vi "BallSequencing.vi"(0 "Balls In Robot":i32, 1 "Speed of Harvester":dbl, 5 "Shoot":bool, 7 "Ball S12 Process":bool, 9 "Ball S3 Process":bool, 11 "Speed of Conveyor":dbl, 12 "SP 1 Triggered":bool, 13 "SP 2 Triggered":bool, 14 "SP 3 Triggered":bool) -> (2 "Conveyer Output":dbl, 3 "Harvester Output":dbl, 4 "Balls In Robot Output":i32, 6 "Shoot Output":bool, 8 "Ball S12 Process Output":bool, 10 "Ball S3 Process Output":bool)   [LabVIEW 2011]
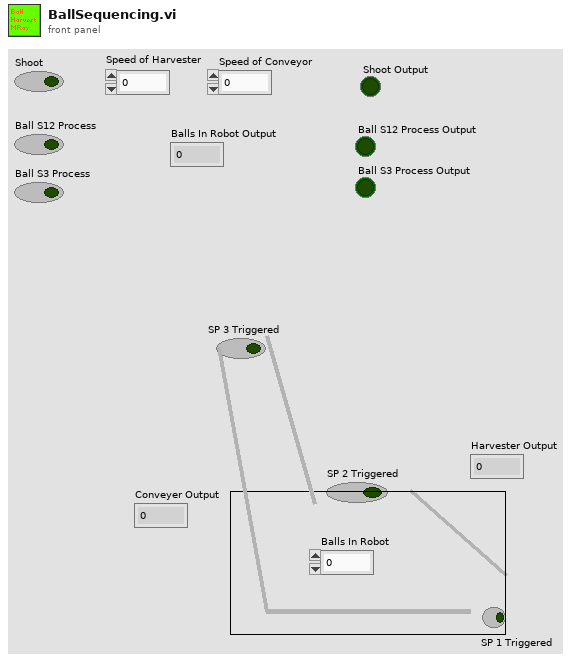
[diagram p1: front panel]
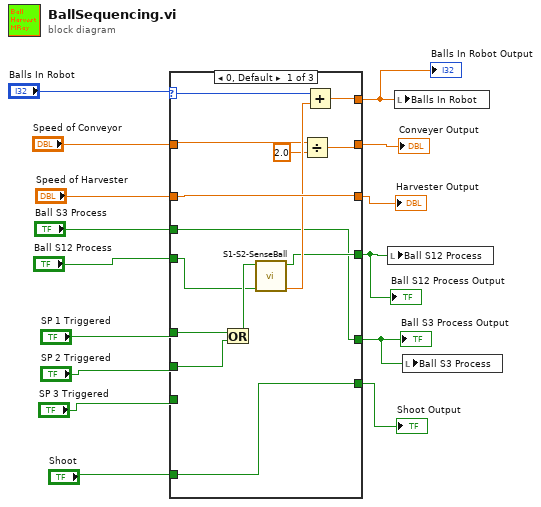
[diagram p0: block diagram]
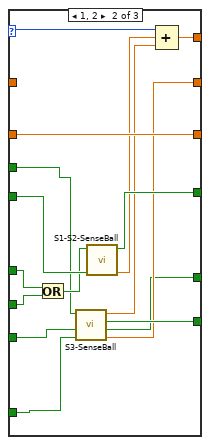
[diagram p2: hidden frame]
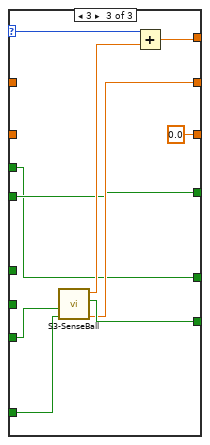
[diagram p3: hidden frame]
diagram:
  n1 = case shown="0, Default" "Balls In Robot" {
    selector: "Balls In Robot" -> [w28 w37 w54]
    tunnel: "SP 1 Triggered" -> [w25 w43 _]
    tunnel: "SP 2 Triggered" -> [w24 w44 _]
    tunnel: [w29 w40 0.0 ("Speed of Harvester")] -> w15
    tunnel: "Speed of Harvester" -> [w29 w40 _]
    tunnel: "Speed of Conveyor" -> [w20 _ _]
    tunnel: [w18 w31 w48] -> w3
    tunnel: [w27 w39 w53] -> w2
    tunnel: "SP 3 Triggered" -> [_ w35 w49]
    tunnel: "Ball S3 Process" -> [w16 w34 w46]
    tunnel: "Ball S12 Process" -> [w22 w45 w47]
    tunnel: [w21 w41 w47] -> w4
    tunnel: "Shoot" -> [w17 w36 w52]
    tunnel: [w17 w33 w51] -> w5
    tunnel: [w16 w30 w46] -> w1
    frame 0, Default {
      n2 = Or(x=w25, y=w24) -> (x .or. y?=w23:bool)
      n3 = call "S1-S2-SenseBall.vi"("Ball in Process in"=w22, "Sense Ball"=w23) -> ("Ball Counter"=w26:dbl, "Ball in Process out"=w21:bool)  [unwired: 8 in]
      n4 = Divide(x=w20, y=2.0) -> (x/y=w18:dbl)
      n5 = Add(x=w28, y=w26) -> (x+y=w27:dbl)
    }
    frame 1, 2 {
      n6 = Or(x=w43, y=w44) -> (x .or. y?=w42:bool)
      n7 = call "S3-SenseBall.vi"("Ball S3 Process"=w34, "Sense Ball"=w35, "Trigger Shooter"=w36) -> ("Ball Counter"=w32:dbl, "Trigger Shooter Output"=w33:bool, "Ball S3 Process Output"=w30:bool, "Conveyer Output"=w31:dbl)  [unwired: 4 in]
      n8 = call "S1-S2-SenseBall.vi"("Ball in Process in"=w45, "Sense Ball"=w42) -> ("Ball Counter"=w38:dbl, "Ball in Process out"=w41:bool)  [unwired: 8 in]
      n9 = Compound Arithmetic op=ADD(w37, w38, w32) -> (w39:dbl)
    }
    frame 3 {
      n10 = call "S3-SenseBall.vi"("Sense Ball"=w49, "Trigger Shooter"=w52) -> ("Ball Counter"=w50:dbl, "Trigger Shooter Output"=w51:bool, "Conveyer Output"=w48:dbl)  [unwired: 5 in, 1 out]
      n11 = Add(x=w54, y=w50) -> (x+y=w53:dbl)
    }
  }
  "Shoot Output" <- w5
  "Ball S12 Process Output" <- w4
  "Harvester Output" <- w15
  "Conveyer Output" <- w3
  "Balls In Robot Output" <- w2
  "Ball S3 Process Output" <- w1
  n12 = local write "Ball S12 Process"(w4) -> ()
  n13 = local write "Balls In Robot"(w2) -> ()
  n14 = local write "Ball S3 Process"(w1) -> ()
